vi "OCT - Auto Power Spectrums.vi"(0 "reference in":refnum<class "GSwFormDSP.lvclass">, 5 "error in (no error)":errorcluster, 7 "Octave Bandwidth":T1(ring)) -> (14 "reference out":refnum<class "GSwFormDSP.lvclass">, 19 "error out":errorcluster)   [LabVIEW 2020, in "GSwFormDSP.lvclass"]
uses:
  GSwFormDSP.lvclass
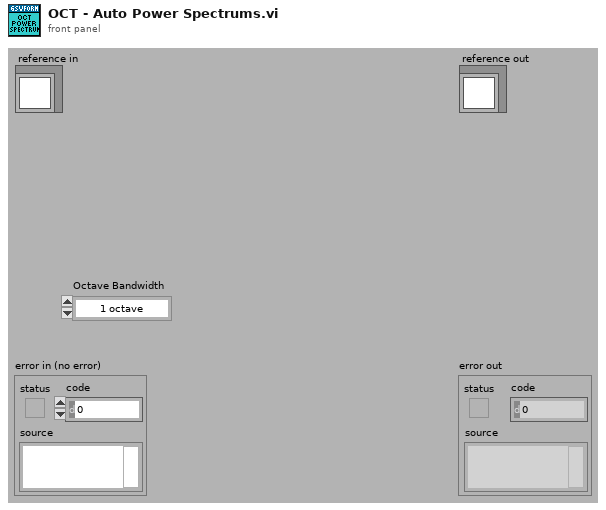
[diagram p1: front panel]
types:
  T1 = enum16{"1 octave", "1/3 octave", "1/6 octave", "1/12 octave", "1/24 octave"}
  T2 = typedef "GSwFormDSP.lvclass/ObjectAttributesRef.ctl" = refnum<data-value>
  T3 = typedef "GSwFormDSP.lvclass/ObjectAttributes.ctl" = cluster{"Wform Ref":refnum<data-value>, "Nb Signals":i32, "Spectral Function Parameters":T4, "FFT":waveform(cdb)[], "Nb FFT":i32, "Nb Averages":i32[], "Reference Indexes":i32[], "Response Indexes":i32[], "Coherence":waveform(dbl)[], "TDF Parameters":T6, "DAQ":cluster{"Duration (sec)":dbl, "Buffer Size (Samples)":i32, "Offset (Samples)":i32}, "Filter Impulse Response (TDF)":waveform(dbl), "Sound Playback":T7}
  T4 = typedef "GSwFormDSP.lvclass/Spectral Parameters.ctl" = cluster{"Frequency resolution (Hz)":dbl, "Overlap":dbl, "Window":T5}
  T5 = typedef "NI_AALPro.lvlib/windowTd.ctl" = u32
  T6 = typedef "GSwFormDSP.lvclass/TDF Parameters.ctl" = cluster{"Filter":enum32{"Lowpass", "Highpass", "Bandpass", "Bandstop"}, "Type:":enum16{"Butterworth", "Chebyshev", "Inv Chebyshev", "Elliptic", "Bessel"}, "LP cutoff freq":dbl, "HP cutoff freq":dbl, "Order":i32, "passband ripple (dB)":dbl, "stopband attenuation (dB)":dbl, "Phaseless Filter":bool, "Include Fade IN and OUT":bool}
  T7 = typedef "GSwFormDSP.lvclass/Sound Playback.ctl" = cluster{"Timer start (ms)":u32, "task ID":T8, "Cursor Init Location (s)":dbl, "SC Volume":dbl}
  T8 = typedef "Sound Output Task ID.ctl" = u32
  T9 = cluster{"low frequency":dbl, "high frequency":dbl}
  T10 = cluster{"nominal frequencies [Hz]":dbl[], "band power":dbl[]}[]
  T11 = typedef "SoundVib_Octave.lvlib/sv_Octave Info.ctl" = cluster{"standard":enum16{"ANSI S.1.11", "IEC 1260"}, "bandwidth":enum16{"1 octave", "1/3 octave", "1/6 octave", "1/12 octave", "1/24 octave"}, "low band":i32, "high band":i32, "weighting filter":T12, "dB reference":dbl, "dB On":bool, "unit label":string, "channel name":string, "description":string, "engineering units":T13, "custom label":string, "spectrum type":enum16{"power", "magnitude"}, "spectral density":bool, "filters settled":bool}
  T12 = typedef "svc_Weighting Filter Text Ring.ctl" = u16
  T13 = typedef "svc_Engineering Units Text Ring.ctl" = u16
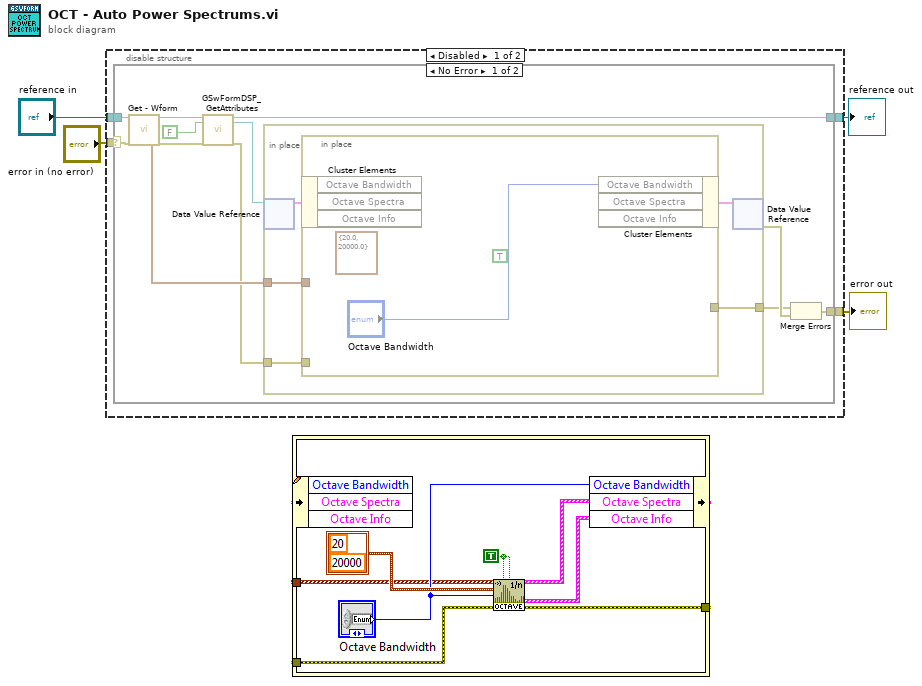
[diagram p0: block diagram]
diagram:
  n1 = disable-structure shown="Disabled" {
    disable-tunnel: "error in (no error)" -> [w8 _]
    disable-tunnel: [w7 _] -> w3
    disable-tunnel: "reference in" -> [w6 _]
    disable-tunnel: [w5 _] -> w1
    frame Disabled {
      n2 = case shown="No Error" w8 {
        selector: w8 -> [w14 w35]
        tunnel: [w20 w35] -> w7
        tunnel: [w17 w34] -> w5
        tunnel: w6 -> [w15 w34]
        frame No Error {
          n3 = call-dynamic "Get - Wform.vi"("reference in"=w15, "error in (no error)"=w14) -> ("wForms"=w11:waveform(dbl)[], "reference out"=w12:refnum<class "GSwFormDSP.lvclass">, "error out"=w13:errorcluster)  [unwired: 15 in]
          n4 = call "GSwFormDSP_GetAttributes.vi"("reference in"=w12, "return data? (T)"=FALSE, "error in (no error)"=w13) -> ("reference out"=w17:refnum<class "GSwFormDSP.lvclass">, "attributes ref"=w16:T2, "error out"=w10:errorcluster)  [unwired: 13 in, 1 out]
          n5 = in-place {
            in-place-border: w11 -> [w23]
            in-place-border: w10 -> [w22]
            in-place-border: [w21] -> w9
            n6 = in-place-dvr #1(w16) -> (w24:T3)  [unwired: 1 out]
            n7 = in-place {
              in-place-border: w23 -> [w33]
              in-place-border: w22 -> [w30]
              in-place-border: [w28] -> w21
              w26 = TRUE ("restart averaging (F)")
              w27 = T9 {"low frequency"=20.0, "high frequency"=20000.0} ("frequency range [Hz]")
              n8 = in-place-cluster #2(w24) -> ()  [unwired: 3 out]
              n9 = in-place-cluster #2("Octave Bandwidth"="Octave Bandwidth") -> (w25:T3, "Octave Spectra"=w32:T10, "Octave Info"=w31:T11[])
            }
            n10 = in-place-dvr #1(w25) -> (w19:errorcluster)  [unwired: 1 out]
          }
          n11 = Merge Errors(w9, w19) -> (w20:errorcluster)
        }
        frame Error {
        }
      }
    }
    frame Enabled {
    }
  }
  "error out" <- w3
  "reference out" <- w1
